vi "Save Config Dialog.vi"(8 "error in (no error)":errorcluster, 11 "Current Config Path":path) -> (0 "error out":errorcluster, 2 "Cancelled":bool, 3 "New Config Path":path)   [LabVIEW 2017, in "File IO.lvlib"]
uses:
  File IO.lvlib
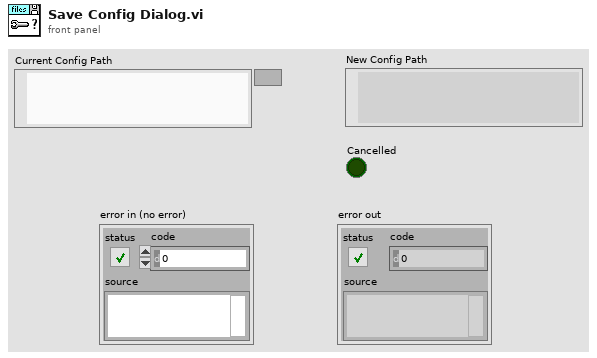
[diagram p1: front panel]
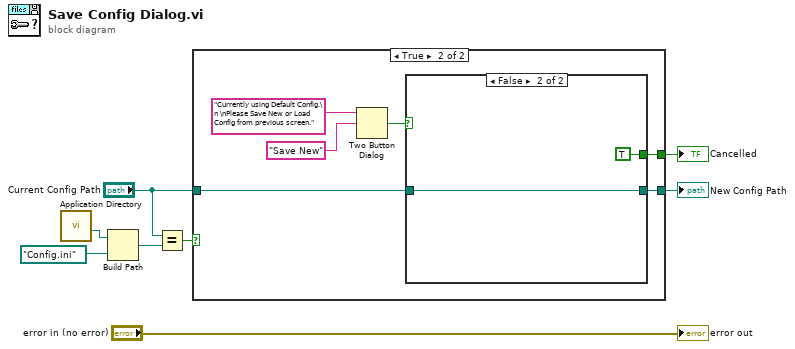
[diagram p0: block diagram]
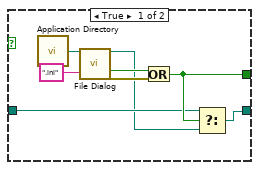
[diagram p3: hidden frame]
diagram:
  n1 = call <vilib>:"Application Directory.vi"() -> ("Application Directory"=w7:path)
  n2 = Build Path(base path=w7, name or relative path=path "Config.ini" ("Error file")) -> (appended path=w1:path)
  n3 = Equal?(x="Current Config Path", y=w1) -> (x = y?=w6:bool)
  n4 = case shown="True" w6 {
    tunnel: "Current Config Path" -> [w9 w14]
    tunnel: [w9 w13] -> w5
    tunnel: [_ w12] -> w4
    frame False {
    }
    frame True {
      n5 = Two Button Dialog(message="Currently using Default Config.\n \nPlease Save New or Load Config from previous screen.", 2:"Save New" ("T button name (\"OK\")")) -> (T button?=w15:bool)  [unwired: 1 in]
      n6 = case shown="False" w15 {
        tunnel: w14 -> [w18 w25]
        tunnel: [w17 w25] -> w13
        tunnel: [w19 TRUE ("cancelled")] -> w12
        frame True {
          n7 = call <vilib>:"Application Directory.vi"() -> ("Application Directory"=w23:path)
          n8 = call "File Dialog"("start path"=w23, "pattern (all files)"=".ini" ("pattern label")) -> ("selected path"=w16:path, "cancelled"=w20:bool, "error out"=w21:errorcluster)  [unwired: 10 in, 1 out]
          n9 = Or(x=w20, y=w21) -> (x .or. y?=w19:bool)
          n10 = Select(t=w18, s=w19, f=w16) -> (s? t:f=w17:path)
        }
        frame False {
        }
      }
    }
  }
  "New Config Path" <- w5
  "Cancelled" <- w4
  "error out" <- "error in (no error)"
